vi "中英文全局-8.6.vi"() -> ()   [LabVIEW 2013]
panel:
  in  "英文?":bool
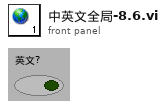
[diagram p1: front panel]
diagram:
